vi "UpdateEngine.vi"(8 "error in (no error)":errorcluster, 11 "Pump_1AI_1DO_2DI in":refnum<class "PM_Group.lvclass">) -> (0 "error out":errorcluster, 3 "Pump_1AI_1DO_2DI out":refnum<class "PM_Group.lvclass">)   [LabVIEW 2019, in "PM_Group.lvclass"]
uses:
  PM_Group.lvclass
  PM_Group.lvclass/PM_Group.ctl
  Sig_DA_class/Sig_DA.lvclass/Sig_DA.ctl
  Proccess_class/Proccess.lvclass/Proccess.ctl
  TypeDef/StatePump.ctl
  subvis/bool_change.vi
  Sig_DA_class/private/write_to_db.vi
  Proccess_class/Read Name.vi
  Proccess_class/Read Logger.vi
  Sig_DA_class/Sig_DA.lvclass
  D:/GIT H4000/H4000/src/Proccess_class/Proccess.lvclass
  Logger_class/WriteEvent.vi
  FPGA_API_class/FPGA API.lvclass
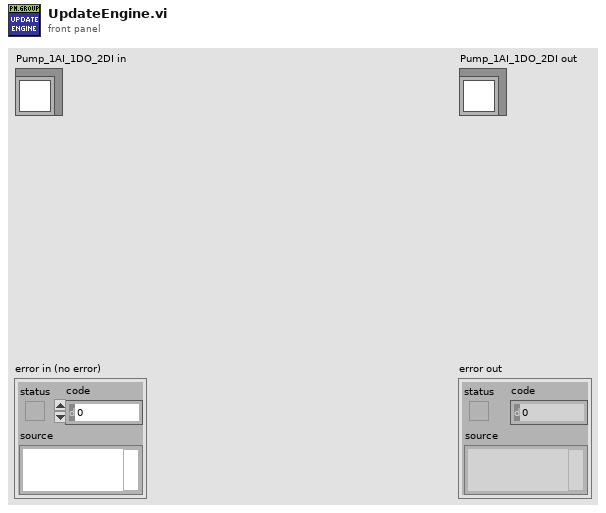
[diagram p1: front panel]
types:
  T1 = typedef "StatePump.ctl" = enum16{"Off", "TupningOn", "On", "TurningOff"}
  T2 = typedef "DI index.ctl" = u8
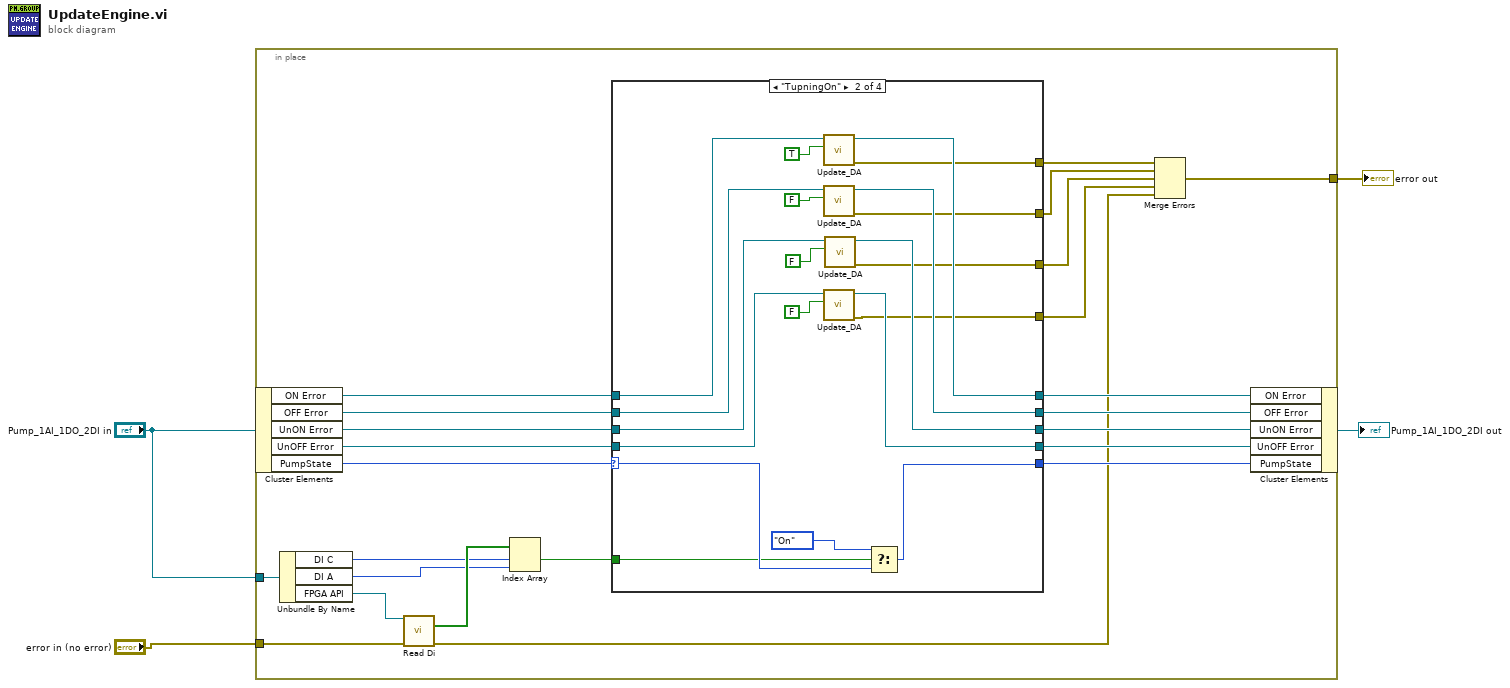
[diagram p0: block diagram]
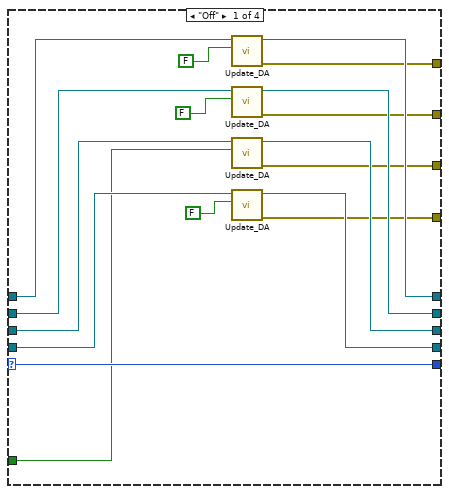
[diagram p2: hidden frame]
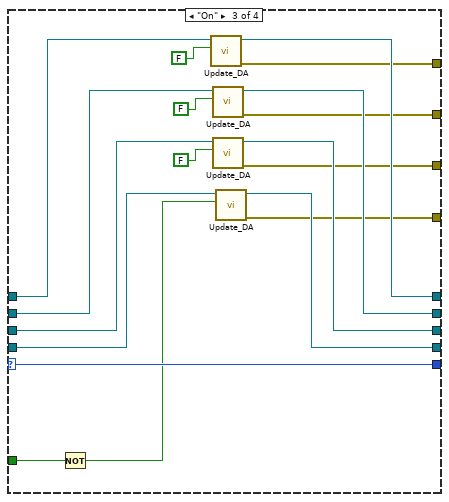
[diagram p3: hidden frame]
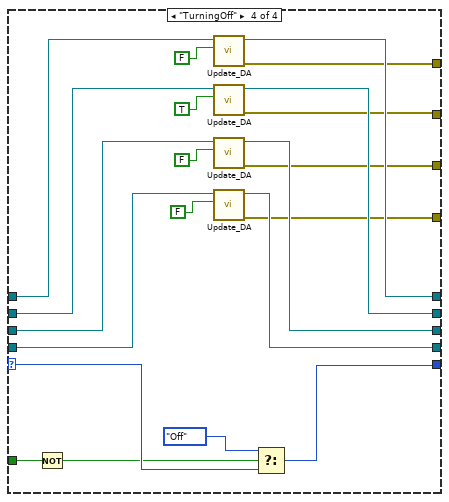
[diagram p4: hidden frame]
diagram:
  n1 = in-place {
    in-place-border: "error in (no error)" -> [w8]
    in-place-border: [w13] -> w3
    in-place-border: "Pump_1AI_1DO_2DI in" -> [w12]
    n2 = in-place-cluster #1("Pump_1AI_1DO_2DI in") -> ("ON Error"=w23:refnum<class "Sig_DA.lvclass">, "OFF Error"=w21:refnum<class "Sig_DA.lvclass">, "UnON Error"=w25:refnum<class "Sig_DA.lvclass">, "UnOFF Error"=w19:refnum<class "Sig_DA.lvclass">, "PumpState"=w27:T1)
    n3 = Unbundle By Name(w12) -> ("DI C"=w10:T2, "DI A"=w9:T2, "FPGA API"=w6:refnum<class "FPGA API.lvclass">)
    n4 = call "Read Di.vi"("FPGA API in"=w6, "error in (no error)"=w8) -> ("DIs"=w11:bool[], "error out"=w5:errorcluster)  [unwired: 11 in, 1 out]
    n5 = Index Array(array=w11, index #1=w10, index #2=w9) -> (element #1=w7:bool)  [unwired: 1 out]
    n6 = case shown="\"TupningOn\"" w27 {
      selector: w27 -> [w44 w64 w82 w103]
      tunnel: [w44 w62 w82 w101] -> w26
      tunnel: w25 -> [w43 w53 w74 w91]
      tunnel: [w39 w60 w79 w97] -> w24
      tunnel: w23 -> [w40 w61 w80 w98]
      tunnel: [w36 w54 w75 w94] -> w22
      tunnel: w21 -> [w37 w55 w76 w95]
      tunnel: [w33 w50 w71 w89] -> w20
      tunnel: w19 -> [w34 w51 w72 w90]
      tunnel: [w42 w52 w73 w88] -> w18
      tunnel: [w32 w46 w66 w84] -> w14
      tunnel: [w31 w47 w67 w85] -> w15
      tunnel: [w30 w48 w68 w87] -> w16
      tunnel: [w29 w49 w69 w86] -> w17
      tunnel: w7 -> [w28 w45 w65 w83]
      frame "Off" {
        n7 = call "Update_DA.vi"("RAW"=FALSE, "Sig_DA in"=w40) -> ("error out"=w29:errorcluster, "Sig_DA out"=w39:refnum<class "Sig_DA.lvclass">)  [unwired: 7 in, 1 out]
        n8 = call "Update_DA.vi"("RAW"=FALSE, "Sig_DA in"=w37) -> ("error out"=w30:errorcluster, "Sig_DA out"=w36:refnum<class "Sig_DA.lvclass">)  [unwired: 7 in, 1 out]
        n9 = call "Update_DA.vi"("RAW"=w28, "Sig_DA in"=w43) -> ("error out"=w31:errorcluster, "Sig_DA out"=w42:refnum<class "Sig_DA.lvclass">)  [unwired: 7 in, 1 out]
        n10 = call "Update_DA.vi"("RAW"=FALSE, "Sig_DA in"=w34) -> ("error out"=w32:errorcluster, "Sig_DA out"=w33:refnum<class "Sig_DA.lvclass">)  [unwired: 7 in, 1 out]
      }
      frame "TupningOn" {
        n11 = call "Update_DA.vi"("RAW"=TRUE, "Sig_DA in"=w61) -> ("error out"=w49:errorcluster, "Sig_DA out"=w60:refnum<class "Sig_DA.lvclass">)  [unwired: 7 in, 1 out]
        n12 = call "Update_DA.vi"("RAW"=FALSE, "Sig_DA in"=w55) -> ("error out"=w48:errorcluster, "Sig_DA out"=w54:refnum<class "Sig_DA.lvclass">)  [unwired: 7 in, 1 out]
        n13 = call "Update_DA.vi"("RAW"=FALSE, "Sig_DA in"=w51) -> ("error out"=w46:errorcluster, "Sig_DA out"=w50:refnum<class "Sig_DA.lvclass">)  [unwired: 7 in, 1 out]
        n14 = call "Update_DA.vi"("RAW"=FALSE, "Sig_DA in"=w53) -> ("error out"=w47:errorcluster, "Sig_DA out"=w52:refnum<class "Sig_DA.lvclass">)  [unwired: 7 in, 1 out]
        n15 = Select(t=StatePump."On", s=w45, f=w64) -> (s? t:f=w62:T1)
      }
      frame "On" {
        n16 = Not(x=w65) -> (.not. x?=w70:bool)
        n17 = call "Update_DA.vi"("RAW"=FALSE, "Sig_DA in"=w80) -> ("error out"=w69:errorcluster, "Sig_DA out"=w79:refnum<class "Sig_DA.lvclass">)  [unwired: 7 in, 1 out]
        n18 = call "Update_DA.vi"("RAW"=FALSE, "Sig_DA in"=w76) -> ("error out"=w68:errorcluster, "Sig_DA out"=w75:refnum<class "Sig_DA.lvclass">)  [unwired: 7 in, 1 out]
        n19 = call "Update_DA.vi"("RAW"=FALSE, "Sig_DA in"=w74) -> ("error out"=w67:errorcluster, "Sig_DA out"=w73:refnum<class "Sig_DA.lvclass">)  [unwired: 7 in, 1 out]
        n20 = call "Update_DA.vi"("RAW"=w70, "Sig_DA in"=w72) -> ("error out"=w66:errorcluster, "Sig_DA out"=w71:refnum<class "Sig_DA.lvclass">)  [unwired: 7 in, 1 out]
      }
      frame "TurningOff" {
        n21 = Not(x=w83) -> (.not. x?=w100:bool)
        n22 = call "Update_DA.vi"("RAW"=FALSE, "Sig_DA in"=w98) -> ("error out"=w86:errorcluster, "Sig_DA out"=w97:refnum<class "Sig_DA.lvclass">)  [unwired: 7 in, 1 out]
        n23 = call "Update_DA.vi"("RAW"=TRUE, "Sig_DA in"=w95) -> ("error out"=w87:errorcluster, "Sig_DA out"=w94:refnum<class "Sig_DA.lvclass">)  [unwired: 7 in, 1 out]
        n24 = call "Update_DA.vi"("RAW"=FALSE, "Sig_DA in"=w91) -> ("error out"=w85:errorcluster, "Sig_DA out"=w88:refnum<class "Sig_DA.lvclass">)  [unwired: 7 in, 1 out]
        n25 = call "Update_DA.vi"("RAW"=FALSE, "Sig_DA in"=w90) -> ("error out"=w84:errorcluster, "Sig_DA out"=w89:refnum<class "Sig_DA.lvclass">)  [unwired: 7 in, 1 out]
        n26 = Select(t=StatePump."Off", s=w100, f=w103) -> (s? t:f=w101:T1)
      }
    }
    n27 = Merge Errors(w17, w16, w15, w14, w5) -> (w13:errorcluster)
    n28 = in-place-cluster #1("ON Error"=w24, "OFF Error"=w22, "UnON Error"=w18, "UnOFF Error"=w20, "PumpState"=w26) -> (→"Pump_1AI_1DO_2DI out":refnum<class "PM_Group.lvclass">)
  }
  "error out" <- w3
